vi "readU64.vi"(8 "error in (no error)":errorcluster, 11 "ModbusBuffer in":refnum<class "ModbusBufferBuilder.lvclass">) -> (0 "error out":errorcluster, 2 "Output":u64, 3 "ModbusBuffer out":refnum<class "ModbusBufferBuilder.lvclass">)   [LabVIEW 2016, in "ModbusBufferBuilder.lvclass"]
uses:
  ModbusBufferBuilder.lvclass
  ModbusBufferBuilder.lvclass/ModbusBufferBuilder.ctl
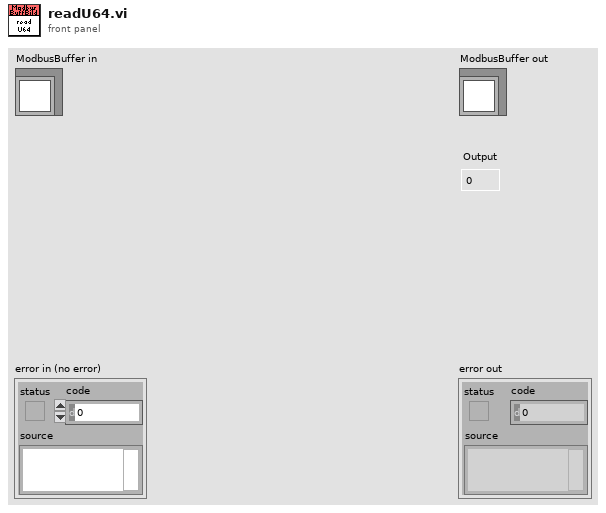
[diagram p1: front panel]
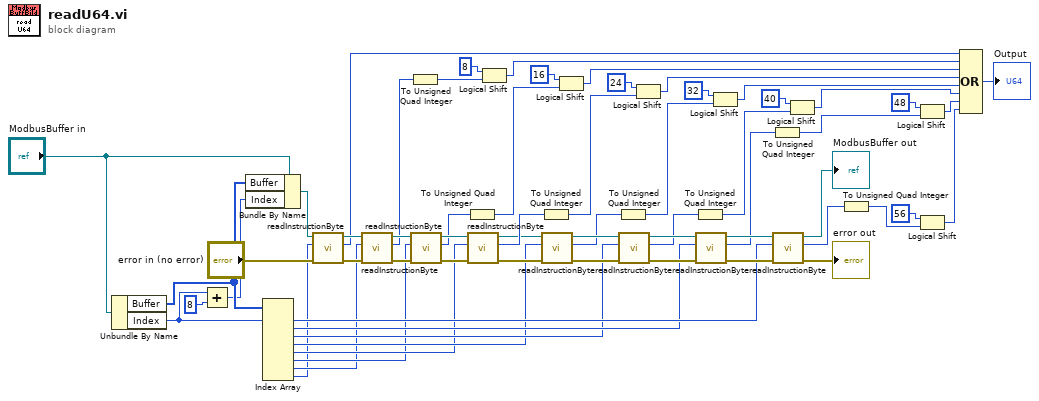
[diagram p0: block diagram]
diagram:
  n1 = Unbundle By Name("ModbusBuffer in") -> ("Buffer"=w60:u16[], "Index"=w57:i32)
  n2 = Add(x=w57, y=8) -> (x+y=w55:i32)
  n3 = Bundle By Name(cluster="ModbusBuffer in", "Buffer"=w60, "Index"=w55) -> (w59:refnum<class "ModbusBufferBuilder.lvclass">)
  n4 = Index Array(array=w60, index #1=w57) -> (element #1=w8:u16, element #2=w7:u16, element #3=w6:u16, element #4=w5:u16, element #5=w4:u16, element #6=w3:u16, element #7=w2:u16, element #8=w1:u16)  [unwired: 7 in]
  n5 = call "readInstructionByte.vi"("error in (no error)"="error in (no error)", "Instruction"=w1, "ModbusBuffer in"=w59) -> ("error out"=w52:errorcluster, "Output"=w53:u8, "ModbusBuffer out"=w54:refnum<class "ModbusBufferBuilder.lvclass">)  [unwired: 6 in]
  n6 = call "readInstructionByte.vi"("error in (no error)"=w52, "Instruction"=w2, "ModbusBuffer in"=w54) -> ("error out"=w46:errorcluster, "Output"=w40:u8, "ModbusBuffer out"=w48:refnum<class "ModbusBufferBuilder.lvclass">)  [unwired: 6 in]
  n7 = To Unsigned Quad Integer(1:w40) -> (0:w39:u64)
  n8 = call "readInstructionByte.vi"("error in (no error)"=w46, "Instruction"=w3, "ModbusBuffer in"=w48) -> ("error out"=w45:errorcluster, "Output"=w38:u8, "ModbusBuffer out"=w47:refnum<class "ModbusBufferBuilder.lvclass">)  [unwired: 6 in]
  n9 = To Unsigned Quad Integer(1:w38) -> (0:w37:u64)
  n10 = call "readInstructionByte.vi"("error in (no error)"=w45, "Instruction"=w4, "ModbusBuffer in"=w47) -> ("error out"=w21:errorcluster, "Output"=w36:u8, "ModbusBuffer out"=w26:refnum<class "ModbusBufferBuilder.lvclass">)  [unwired: 6 in]
  n11 = Logical Shift(y=i16 8, x=w39) -> (x << y=w50:u64)
  n12 = To Unsigned Quad Integer(1:w36) -> (0:w35:u64)
  n13 = call "readInstructionByte.vi"("error in (no error)"=w21, "Instruction"=w5, "ModbusBuffer in"=w26) -> ("error out"=w20:errorcluster, "Output"=w16:u8, "ModbusBuffer out"=w25:refnum<class "ModbusBufferBuilder.lvclass">)  [unwired: 6 in]
  n14 = Logical Shift(y=i16 16, x=w37) -> (x << y=w41:u64)
  n15 = To Unsigned Quad Integer(1:w16) -> (0:w34:u64)
  n16 = call "readInstructionByte.vi"("error in (no error)"=w20, "Instruction"=w6, "ModbusBuffer in"=w25) -> ("error out"=w19:errorcluster, "Output"=w15:u8, "ModbusBuffer out"=w24:refnum<class "ModbusBufferBuilder.lvclass">)  [unwired: 6 in]
  n17 = Logical Shift(y=i16 24, x=w35) -> (x << y=w42:u64)
  n18 = To Unsigned Quad Integer(1:w15) -> (0:w31:u64)
  n19 = call "readInstructionByte.vi"("error in (no error)"=w19, "Instruction"=w7, "ModbusBuffer in"=w24) -> ("error out"=w18:errorcluster, "Output"=w14:u8, "ModbusBuffer out"=w23:refnum<class "ModbusBufferBuilder.lvclass">)  [unwired: 6 in]
  n20 = Logical Shift(y=i16 32, x=w34) -> (x << y=w12:u64)
  n21 = To Unsigned Quad Integer(1:w14) -> (0:w30:u64)
  n22 = call "readInstructionByte.vi"("error in (no error)"=w18, "Instruction"=w8, "ModbusBuffer in"=w23) -> ("error out"=→"error out":errorcluster, "Output"=w13:u8, "ModbusBuffer out"=→"ModbusBuffer out":refnum<class "ModbusBufferBuilder.lvclass">)  [unwired: 6 in]
  n23 = Logical Shift(y=i16 40, x=w31) -> (x << y=w11:u64)
  n24 = To Unsigned Quad Integer(1:w13) -> (0:w27:u64)
  n25 = Logical Shift(y=i16 48, x=w30) -> (x << y=w10:u64)
  n26 = Logical Shift(y=i16 56, x=w27) -> (x << y=w9:u64)
  n27 = Compound Arithmetic op=OR(w53, w50, w41, w42, w12, w11, w10, w9) -> (→"Output":u64)
